vi "Request Spawn.vi"(9 "Number of Requests":i32, 10 "Request Queue":refnum<queue>, 11 "Caller Return Queue":refnum<queue>) -> ()   [LabVIEW 2019, in "Network Interface.lvlib" / "Network Session Handler.lvclass"]
uses:
  <vilib>/gpm_packages/@cs/Network-Sink/Source/Network Interface/Network Session Handler/Network Session Handler.lvclass
  <vilib>/Utility/error.llb/Error Cluster From Error Code.vi
  <vilib>/ErrorRing/Error Ring.xnode
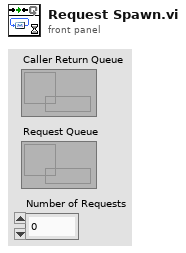
[diagram p1: front panel]
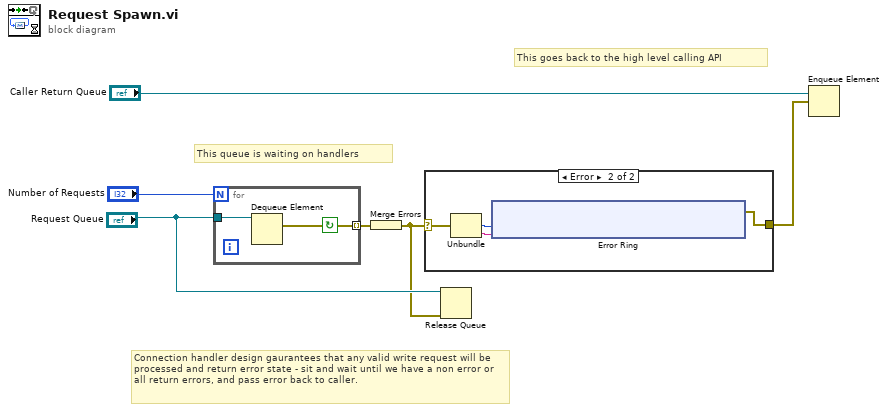
[diagram p0: block diagram]
diagram:
  # "This queue is waiting on handlers"
  # "This goes back to the high level calling API"
  # "Connection handler design gaurantees that any valid write request will be processed and return error state - sit and wait until we have a non error or all return errors, and pass error back to caller."
  n1 = for {
    N: "Number of Requests" -> [_]
    tunnel: "Request Queue" -> [w8]
    tunnel: [w7] -> w2 mode=indexing
    stop <- w7 continue-if-true
    n2 = Dequeue Element(queue=w8) -> (element=w7:errorcluster)  [unwired: 2 in, 3 out]
  }
  n3 = Merge Errors(w2) -> (w1:errorcluster)
  n4 = case shown="Error" w1 {
    selector: w1 -> [w9 w13]
    tunnel: [w9 w10] -> w4
    frame No Error {
    }
    frame Error {
      n5 = Unbundle(w13) -> ("code"=w12:i32, "source"=w11:string)  [unwired: 1 out]
      n6 = xnode "Error Ring"("parameter 0"=w12, "parameter 1"=w11) -> ("error out"=w10:errorcluster)
    }
  }
  n7 = Release Queue(queue="Request Queue", error in (no error)=w1) -> ()  [unwired: 1 in, 3 out]
  n8 = Enqueue Element(queue="Caller Return Queue", element=w4) -> ()  [unwired: 2 in, 3 out]
